vi "GetOrMakeSpecialization.vi"(5 "Extra Scripting (None)":refnum<vi>, 7 "App":refnum<vi>, 8 "Element Type":variant, 9 "Specialized Name Root":string, 10 "Specialized Folder":path, 11 "Template Library/Class":path) -> (0 "error out":errorcluster, 3 "Specialized Instance Path":path)   [LabVIEW 2020, in "FlexBlocks.lvlib"]
uses:
  FlexBlocks.lvlib
  <resource>/ChannelSupport/_ChannelScriptingSupport/_ChannelScriptingSupport.lvlib
panel:
  in  "Force Update? (F)":bool
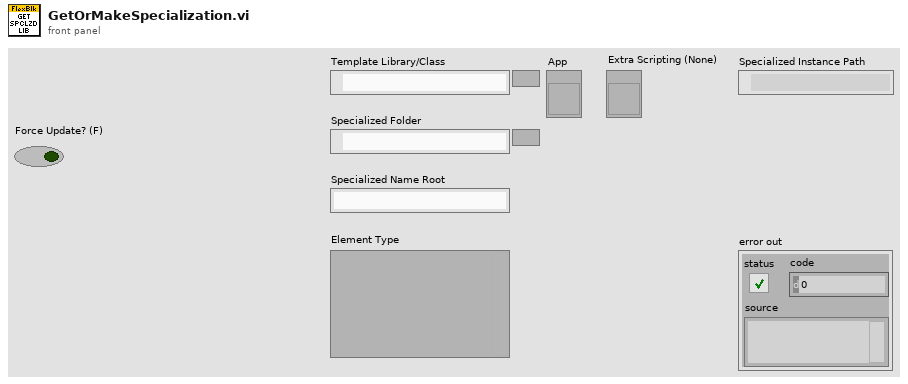
[diagram p1: front panel]
types:
  T1 = typedef "_ChannelScriptingSupport.lvlib/ElementControlInfo.ctl" = cluster{"projItem":refnum<vi>, "eltCtlPath":path, "eltCtlRef":refnum<vi>}
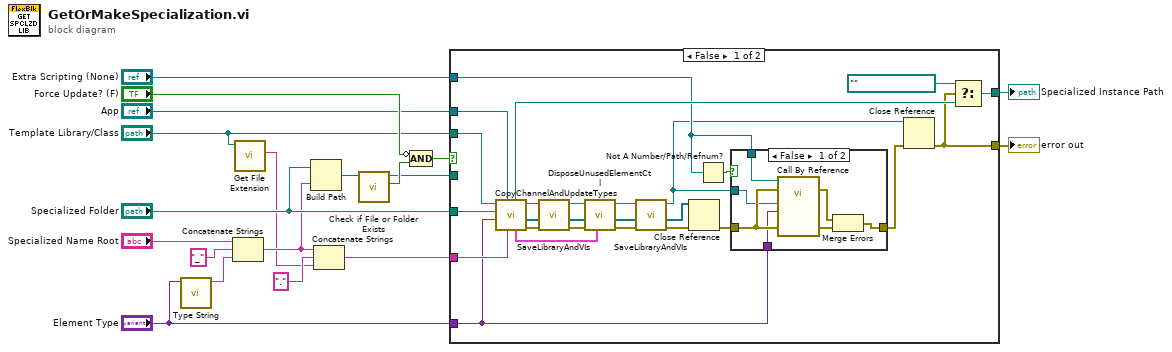
[diagram p0: block diagram]
diagram:
  n1 = call "Type String.vi"("Type"="Element Type") -> ("Type String"=w2:string)  [unwired: 10 in]
  n2 = Concatenate Strings("Specialized Name Root", "_" ("string"), w2) -> (w10:string)
  n3 = call <vilib>:"Get File Extension.vi"("file"="Template Library/Class") -> ("lowercase file extension"=w7:string)  [unwired: 6 in, 4 out]
  n4 = Build Path(base path="Specialized Folder", name or relative path=w10) -> (appended path=w19:path)
  n5 = Concatenate Strings(w10, "." ("string"), w7) -> (w6:string)
  n6 = call <vilib>:"Check if File or Folder Exists.vi"("path"=w19) -> ("file or folder exists?"=w18:bool, "dup path"=w17:path)  [unwired: 8 in, 1 out]
  n7 = Compound Arithmetic op=AND(invert "Force Update? (F)", w18) -> (w16:bool)
  n8 = case shown="False" w16 {
    tunnel: "Template Library/Class" -> [w36 _]
    tunnel: "App" -> [w32 _]
    tunnel: [w23 w54] -> w4
    tunnel: "Specialized Folder" -> [w34 _]
    tunnel: w6 -> [w33 _]
    tunnel: w17 -> [_ w54]
    tunnel: "Element Type" -> [w20 _]
    tunnel: "Extra Scripting (None)" -> [w27 _]
    tunnel: [w22 _] -> w3
    frame False {
      n9 = call <resource>:"CopyChannelAndUpdateTypes.vi"("new library name"=w33, "App"=w32, "elt type"=w20, "new library folder"=w34, "source library path"=w36) -> ("error out"=w44:errorcluster, "vi refs in library"=w40:refnum<vi>[], "copied library"=w45:refnum<vi>, "element control info"=w39:T1, "copied library path"=w35:path)  [unwired: 1 in, 1 out]
      n10 = call <resource>:"SaveLibraryAndVIs.vi"("error in (no error)"=w44, "vi refs in library"=w40, "LVLibrary in"=w45) -> ("error out"=w29:errorcluster, "vi refs in library out"=w30:refnum<vi>[], "LVLibrary out"=w31:refnum<vi>)  [unwired: 6 in]
      n11 = call <resource>:"DisposeUnusedElementCtl.vi"("element control info"=w39, "error in (no error)"=w29, "vi refs in library"=w30, "Library in"=w31) -> ("error out"=w42:errorcluster, "vi refs in library out"=w41:refnum<vi>[], "Library out"=w43:refnum<vi>)  [unwired: 5 in]
      n12 = call <resource>:"SaveLibraryAndVIs.vi"("error in (no error)"=w42, "vi refs in library"=w41, "LVLibrary in"=w43) -> ("error out"=w38:errorcluster, "vi refs in library out"=w37:refnum<vi>[], "LVLibrary out"=w25:refnum<vi>)  [unwired: 6 in]
      n13 = Close Reference(reference=w37, error in (no error)=w38) -> (error out=w26:errorcluster)
      n14 = Not A Number/Path/Refnum?(number/path/refnum=w27) -> (NaN/Path/Refnum?=w28:bool)
      n15 = case shown="False" w28 {
        tunnel: w25 -> [w50 _]
        tunnel: w27 -> [w52 _]
        tunnel: w26 -> [w51 w53]
        tunnel: w20 -> [w49 _]
        tunnel: [w46 w53] -> w24
        frame False {
          n16 = call-by-ref "?"(reference=w52, error in=w51, 8:"error in (no error)"=w51, "Element Type"=w49, "LVLibrary in"=w50) -> (error out=w47:errorcluster, 0:"error out"=w48:errorcluster)  [unwired: 8 in, 1 out]
          n17 = Merge Errors(w47, w48) -> (w46:errorcluster)
        }
        frame True {
        }
      }
      n18 = Close Reference(reference=w25, error in (no error)=w24) -> (error out=w22:errorcluster)
      n19 = Select(t=path "", s=w22, f=w35) -> (s? t:f=w23:path)
    }
    frame True {
      # "Already exists, return path"
    }
  }
  "Specialized Instance Path" <- w4
  "error out" <- w3
